vi "SwerveDrive.vi"   [LabVIEW 2019]
doc: "This VI runs in parallel to other tasks. It can contain as many user-defined periodic loops as you need. These can carry out PID or other sorts of timed response."
uses:
  <vilib>/Rock Robotics/WPI/ThirdParty/Phoenix-LabVIEW/Motor Controller/Controls/CTRE_Phoenix_MotorControl_ControlMode.ctl
  <vilib>/Rock Robotics/WPI/Utilities/WPI_GetSetVariantRefNum.vi
  <vilib>/Rock Robotics/Network Tables/NT Read Numeric Array.vi
  <vilib>/Rock Robotics/Network Tables/NT Write Numeric Array.vi
  Program Files/navX.Library.v2/navX Library v2/navX Library v2.lvlib
types:
  T1 = typedef "WPI_AnalogChannelDevRef.ctl" = cluster{"DevStatus":errorcluster, "Analog Channel":T2}
  T2 = typedef "FPGA_AIChannel.ctl" = enum8{"AI 0", "AI 1", "AI 2", "AI 3", "AI MXP 0", "AI MXP 1", "AI MXP 2", "AI MXP 3", "Invalid"}
  T3 = typedef "WPI_JoystickDevRef.ctl" = cluster{"Device":T4}
  T4 = typedef "WPI_JoystickDeviceEnum.ctl" = enum16{"USB 0", "USB 1", "USB 2", "USB 3", "USB 4", "USB 5"}
  T5 = typedef "WPI_MotorControlDeviceRef.ctl" = cluster{"DeviceStatus":errorcluster, "Type":T6, "PWM":cluster{"PWM Channel":T7, "DeadBand":T8}, "CAN":cluster{"Device Number":u8, "SetOutput VI Ref":variant, "GetOutput VI Ref":variant, "Enable VI Ref":variant, "Disable VI Ref":variant, "Data":variant}, "Invert":bool, "DIO PWM":cluster{"PWM \"Enable\" Channel":T7, "DIOChannel":T9, "PWM Rate":dbl}}
  T6 = typedef "WPI_MotorControlType.ctl" = enum16{"PWM", "CAN", "DIO PWM"}
  T7 = typedef "FPGA_DIOPWMChannel.ctl" = enum8{"PWM 0", "PWM 1", "PWM 2", "PWM 3", "PWM 4", "PWM 5", "PWM 6", "PWM 7", "PWM 8", "PWM 9", "PWM MXP 0", "PWM MXP 1", "PWM MXP 2", "PWM MXP 3", "PWM MXP 4", "PWM MXP 5", "PWM MXP 6", "PWM MXP 7", "PWM MXP 8", "PWM MXP 9", "Invalid"}
  T8 = typedef "WPI_PWMDeadband.ctl" = cluster{"Name":string, "maxPositivePwm":i32, "minPositivePwm":i32, "centerPwm":i32, "maxNegativePwm":i32, "minNegativePwm":i32, "angularRange":u16}
  T9 = typedef "FPGA_DIOChannel.ctl" = enum8{"DIO 0", "DIO 1", "DIO 2", "DIO 3", "DIO 4", "DIO 5", "DIO 6", "DIO 7", "DIO 8", "DIO 9", "DIO MXP 0", "DIO MXP 1", "DIO MXP 2", "DIO MXP 3", "DIO MXP 4", "DIO MXP 5", "DIO MXP 6", "DIO MXP 7", "DIO MXP 8", "DIO MXP 9", "DIO MXP 10", "DIO MXP 11", "DIO MXP 12", "DIO MXP 13", "DIO MXP 14", "DIO MXP 15", "SPI Port CS1", "SPI Port CS2", "SPI Port CS3", "SPI Port MISO", "SPI Port MOSI", "Invalid"}
  T10 = cluster{"PhoenixMotorControlDevRef":T5, "PhoenixMotorControlDevRef":T5, "PhoenixMotorControlDevRef":T5, "PhoenixMotorControlDevRef":T5}
  T11 = typedef "CTRE_Phoenix_MotorControl_ControlMode.ctl" = u16
  T12 = typedef "navX Library v2.lvlib/Z900_navX_DeviceTypeDef.ctl" = cluster{"Interface":cluster{"Protocol":T13, "Update Rate (4Hz-100Hz)":u8, "navX Open TypeDef":variant}, "Notify Packet":refnum<notifier>, "Loop VI Refnum":refnum<vi>, "Ready to Close Occurrence Refnum":refnum<k4>}
  T13 = typedef "navX Library v2.lvlib/Z900_navX_ProtocolTypeDef.ctl" = enum16{"SERIAL", "I2C", "SPI"}
  T14 = cluster{"Yaw":dbl, "Roll":dbl, "Pitch":dbl, "Heading":dbl, "Fused Heading":dbl}
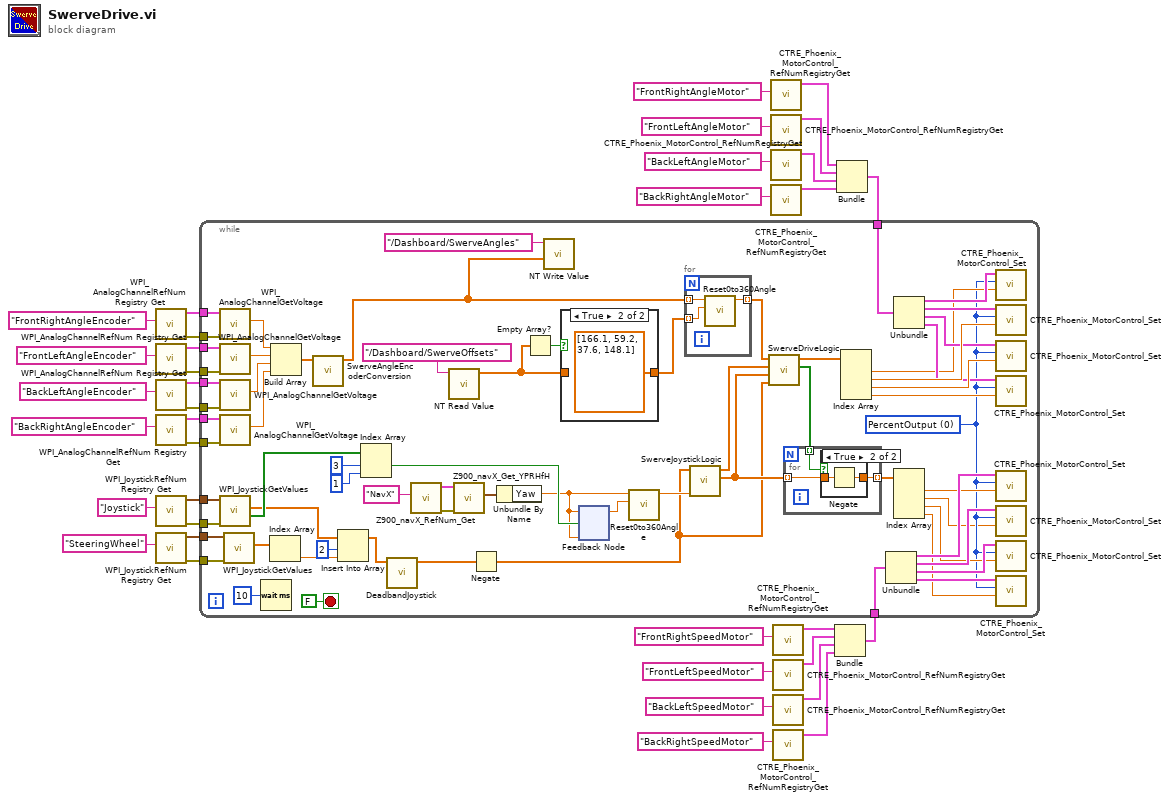
[diagram p0: block diagram]
diagram:
  n1 = call <vilib>:"WPI_AnalogChannelRefNum Registry Get.vi"("refnum name"="FrontRightAngleEncoder") -> ("error out"=w12:errorcluster, "AIDeviceRef"=w22:T1)  [unwired: 9 in]
  n2 = call <vilib>:"WPI_AnalogChannelRefNum Registry Get.vi"("refnum name"="FrontLeftAngleEncoder") -> ("error out"=w11:errorcluster, "AIDeviceRef"=w21:T1)  [unwired: 9 in]
  n3 = call <vilib>:"WPI_AnalogChannelRefNum Registry Get.vi"("refnum name"="BackLeftAngleEncoder") -> ("error out"=w10:errorcluster, "AIDeviceRef"=w20:T1)  [unwired: 9 in]
  n4 = call <vilib>:"WPI_AnalogChannelRefNum Registry Get.vi"("refnum name"="BackRightAngleEncoder") -> ("error out"=w9:errorcluster, "AIDeviceRef"=w19:T1)  [unwired: 9 in]
  n5 = call <vilib>:"WPI_JoystickRefNum Registry Get.vi"("refnum name"="Joystick") -> ("error out"=w4:errorcluster, "JoystickDevRef"=w5:T3)  [unwired: 1 in, 8 out]
  n6 = call <vilib>:"WPI_JoystickRefNum Registry Get.vi"("refnum name"="SteeringWheel") -> ("error out"=w2:errorcluster, "JoystickDevRef"=w3:T3)  [unwired: 1 in, 8 out]
  n7 = call <vilib>:"CTRE_Phoenix_MotorControl_RefNumRegistryGet.vi"("refnum name"="FrontRightAngleMotor") -> ("PhoenixMotorControlDevRef"=w13:T5)  [unwired: 9 in, 1 out]
  n8 = call <vilib>:"CTRE_Phoenix_MotorControl_RefNumRegistryGet.vi"("refnum name"="FrontLeftAngleMotor") -> ("PhoenixMotorControlDevRef"=w17:T5)  [unwired: 9 in, 1 out]
  n9 = call <vilib>:"CTRE_Phoenix_MotorControl_RefNumRegistryGet.vi"("refnum name"="BackLeftAngleMotor") -> ("PhoenixMotorControlDevRef"=w18:T5)  [unwired: 9 in, 1 out]
  n10 = call <vilib>:"CTRE_Phoenix_MotorControl_RefNumRegistryGet.vi"("refnum name"="BackRightAngleMotor") -> ("PhoenixMotorControlDevRef"=w15:T5)  [unwired: 9 in, 1 out]
  n11 = call <vilib>:"CTRE_Phoenix_MotorControl_RefNumRegistryGet.vi"("refnum name"="FrontRightSpeedMotor") -> ("PhoenixMotorControlDevRef"=w16:T5)  [unwired: 9 in, 1 out]
  n12 = call <vilib>:"CTRE_Phoenix_MotorControl_RefNumRegistryGet.vi"("refnum name"="FrontLeftSpeedMotor") -> ("PhoenixMotorControlDevRef"=w1:T5)  [unwired: 9 in, 1 out]
  n13 = call <vilib>:"CTRE_Phoenix_MotorControl_RefNumRegistryGet.vi"("refnum name"="BackLeftSpeedMotor") -> ("PhoenixMotorControlDevRef"=w23:T5)  [unwired: 9 in, 1 out]
  n14 = call <vilib>:"CTRE_Phoenix_MotorControl_RefNumRegistryGet.vi"("refnum name"="BackRightSpeedMotor") -> ("PhoenixMotorControlDevRef"=w24:T5)  [unwired: 9 in, 1 out]
  n15 = Bundle("PhoenixMotorControlDevRef"=w16, "PhoenixMotorControlDevRef"=w1, "PhoenixMotorControlDevRef"=w23, "PhoenixMotorControlDevRef"=w24) -> (w8:T10)  [unwired: 1 in]
  n16 = Bundle("PhoenixMotorControlDevRef"=w13, "PhoenixMotorControlDevRef"=w17, "PhoenixMotorControlDevRef"=w18, "PhoenixMotorControlDevRef"=w15) -> (w14:T10)  [unwired: 1 in]
  n17 = while {
    tunnel: w22 -> [w79]
    tunnel: w21 -> [w74]
    tunnel: w20 -> [w71]
    tunnel: w19 -> [w77]
    tunnel: w14 -> [w87]
    tunnel: w12 -> [w80]
    tunnel: w11 -> [w73]
    tunnel: w10 -> [w70]
    tunnel: w9 -> [w76]
    tunnel: w8 -> [w65]
    tunnel: w5 -> [w61]
    tunnel: w4 -> [w60]
    tunnel: w3 -> [w59]
    tunnel: w2 -> [w58]
    stop <- FALSE stop-if-true
    w81 = T11 0 items=["PercentOutput"=0, "Position"=1, "Velocity"=2, "Current"=3, "Follower"=5, "MotionProfile"=6, "MotionMagic"=7, "MotionProfileArc"=10, "Disabled"=15] ("Control Mode")
    n18 = call <vilib>:"WPI_AnalogChannelGetVoltage.vi"("error in (no error)"=w80, "AIDeviceRef"=w79) -> ("Voltage"=w78:dbl)  [unwired: 7 in, 2 out]
    n19 = call <vilib>:"WPI_AnalogChannelGetVoltage.vi"("error in (no error)"=w73, "AIDeviceRef"=w74) -> ("Voltage"=w72:dbl)  [unwired: 7 in, 2 out]
    n20 = call <vilib>:"WPI_AnalogChannelGetVoltage.vi"("error in (no error)"=w70, "AIDeviceRef"=w71) -> ("Voltage"=w69:dbl)  [unwired: 7 in, 2 out]
    n21 = call <vilib>:"WPI_AnalogChannelGetVoltage.vi"("error in (no error)"=w76, "AIDeviceRef"=w77) -> ("Voltage"=w75:dbl)  [unwired: 7 in, 2 out]
    n22 = call <vilib>:"WPI_JoystickGetValues.vi"("error in (no error)"=w60, "JoystickDevRef"=w61) -> ("Buttons"=w64:bool[], "Axes"=w51:dbl[])  [unwired: 5 in, 3 out]
    n23 = call <vilib>:"WPI_JoystickGetValues.vi"("error in (no error)"=w58, "JoystickDevRef"=w59) -> ("Axes"=w50:dbl[])  [unwired: 5 in, 4 out]
    n24 = Wait (ms)(milliseconds to wait=u32 10) -> ()  [unwired: 1 out]
    n25 = Index Array(array=w50) -> (element=w49:dbl)  [unwired: 1 in]
    n26 = Build Array(w78, w72, w69, w75) -> (w86:dbl[])
    n27 = call "SwerveAngleEncoderConversion.vi"("Voltages"=w86) -> ("Angles"=w52:dbl[])  [unwired: 10 in]
    n28 = Insert Into Array(array=w51, index=2, new element=w49) -> (w47:dbl[])
    n29 = Index Array(array=w64, index #1=3 ("index"), index #2=1 ("index")) -> (element #1=w40:bool)  [unwired: 1 out]
    n30 = call "DeadbandJoystick.vi"("InputArray"=w47) -> ("OutputArray"=w38:dbl[])  [unwired: 10 in]
    n31 = call "Z900_navX_RefNum_Get.vi"("refnum name"="NavX") -> ("error out"=w43:errorcluster, "navX Device"=w44:T12)  [unwired: 9 in]
    n32 = call-poly <vilib>:"NT Read Value.vi"("Name"="/Dashboard/SwerveOffsets") -> ("Numeric Array"=w57:dbl[])  [unwired: 9 in, 1 out]
    n33 = call "Z900_navX_Get_YPRHfH.vi"("error in (no error)"=w43, "navX Device"=w44) -> ("YRPHfH"=w66:T14)  [unwired: 6 in, 3 out]
    n34 = Negate(x=w38) -> (-x=w37:dbl[])
    n35 = Unbundle By Name(w66) -> ("Yaw"=w39:dbl)
    n36 = Empty Array?(array=w57) -> (empty?=w56:bool)
    n37 = call-poly <vilib>:"NT Write Value.vi"("Numeric Array"=w52, "Name"="/Dashboard/SwerveAngles") -> ()  [unwired: 9 in, 1 out]
    n38 = case shown="True" w56 {
      tunnel: [w105 dbl[] [166.1, 59.2, 37.6, 148.1] ("Numeric Array")] -> w55
      tunnel: w57 -> [w105 _]
      frame False {
      }
      frame True {
      }
    }
    n39 = feedback-in #1(w39, w40) -> ()
    n40 = feedback #1(w39) -> (w42:dbl)
    n41 = call "Reset0to360Angle.vi"("Offset"=w42, "AngleInput"=w39) -> ("AngleOutput"=w41:dbl)  [unwired: 9 in]
    n42 = for {
      tunnel: w52 -> [w108] mode=indexing
      tunnel: [w109] -> w92 mode=indexing
      tunnel: w55 -> [w107] mode=indexing
      n43 = call "Reset0to360Angle.vi"("Offset"=w107, "AngleInput"=w108) -> ("AngleOutput"=w109:dbl)  [unwired: 9 in]
    }
    n44 = call "SwerveJoystickLogic.vi"("Gyro"=w41, "Joystick Axes"=w37) -> ("Speeds"=w45:dbl[], "Angles"=w91:dbl[])  [unwired: 7 in]
    n45 = call "SwerveDriveLogic.vi"("Joystick Axes"=w37, "Speeds"=w45, "AngleSetpoints"=w91, "AngleEncoders"=w92) -> ("AngleMotorsReversed"=w93:bool[], "AngleMotorOutputs"=w90:dbl[])  [unwired: 6 in]
    n46 = for {
      tunnel: w45 -> [w111] mode=indexing
      tunnel: [w112] -> w98 mode=indexing
      tunnel: w93 -> [w110] mode=indexing
      n47 = case shown="True" w110 {
        tunnel: w111 -> [w113 w115]
        tunnel: [w113 w114] -> w112
        frame False {
        }
        frame True {
          n48 = Negate(x=w115) -> (-x=w114:dbl)
        }
      }
    }
    n49 = Index Array(array=w90) -> (element #1=w84:dbl, element #2=w103:dbl, element #3=w102:dbl, element #4=w85:dbl)  [unwired: 4 in]
    n50 = Unbundle(w65) -> ("PhoenixMotorControlDevRef"=w89:T5, "PhoenixMotorControlDevRef"=w97:T5, "PhoenixMotorControlDevRef"=w96:T5, "PhoenixMotorControlDevRef"=w95:T5)
    n51 = Unbundle(w87) -> ("PhoenixMotorControlDevRef"=w101:T5, "PhoenixMotorControlDevRef"=w100:T5, "PhoenixMotorControlDevRef"=w99:T5, "PhoenixMotorControlDevRef"=w94:T5)
    n52 = Index Array(array=w98) -> (element #1=w83:dbl, element #2=w67:dbl, element #3=w82:dbl, element #4=w68:dbl)  [unwired: 4 in]
    n53 = call <vilib>:"CTRE_Phoenix_MotorControl_Set.vi"("Output"=w84, "Control Mode"=w81, "PhoenixMotorControlDevRef"=w101) -> ()  [unwired: 7 in, 2 out]
    n54 = call <vilib>:"CTRE_Phoenix_MotorControl_Set.vi"("Output"=w103, "Control Mode"=w81, "PhoenixMotorControlDevRef"=w100) -> ()  [unwired: 7 in, 2 out]
    n55 = call <vilib>:"CTRE_Phoenix_MotorControl_Set.vi"("Output"=w102, "Control Mode"=w81, "PhoenixMotorControlDevRef"=w99) -> ()  [unwired: 7 in, 2 out]
    n56 = call <vilib>:"CTRE_Phoenix_MotorControl_Set.vi"("Output"=w85, "Control Mode"=w81, "PhoenixMotorControlDevRef"=w94) -> ()  [unwired: 7 in, 2 out]
    n57 = call <vilib>:"CTRE_Phoenix_MotorControl_Set.vi"("Output"=w83, "Control Mode"=w81, "PhoenixMotorControlDevRef"=w89) -> ()  [unwired: 7 in, 2 out]
    n58 = call <vilib>:"CTRE_Phoenix_MotorControl_Set.vi"("Output"=w67, "Control Mode"=w81, "PhoenixMotorControlDevRef"=w97) -> ()  [unwired: 7 in, 2 out]
    n59 = call <vilib>:"CTRE_Phoenix_MotorControl_Set.vi"("Output"=w82, "Control Mode"=w81, "PhoenixMotorControlDevRef"=w96) -> ()  [unwired: 7 in, 2 out]
    n60 = call <vilib>:"CTRE_Phoenix_MotorControl_Set.vi"("Output"=w68, "Control Mode"=w81, "PhoenixMotorControlDevRef"=w95) -> ()  [unwired: 7 in, 2 out]
  }
